vi "Accelerometre 1.vi"() -> ()   [LabVIEW 2019]
uses:
  <vilib>/myRIO/Express VI/Onboard Devices/Accelerometer/Accelerometer Express VI.xnode
  <vilib>/myRIO/Instrument Drivers/Onboard Devices/Accelerometer/vis/Read.vi
  <vilib>/myRIO/Instrument Drivers/Onboard Devices/Accelerometer/Accelerometer.lvlib
  <vilib>/myRIO/Common/Instrument Driver Framework/myRIO v1.0/Accelerometer/typedefs/Accelerometer Channels Enum.ctl
  <vilib>/myRIO/Common/Instrument Driver Framework/myRIO v1.0/Accelerometer/typedefs/Accelerometer Channels List.ctl
  <vilib>/myRIO/Common/Instrument Driver Framework/Utilities/typedefs/Generic FPGA Reference.ctl
  <vilib>/myRIO/Common/Instrument Driver Framework/Utilities/typedefs/myRIO v1.0 Reference.ctl
  <vilib>/myRIO/Common/Instrument Driver Framework/Utilities/typedefs/Hardware Version Enum.ctl
  <vilib>/myRIO/Common/Instrument Driver Framework/Utilities/typedefs/myRIO Generic Hardware Reference.ctl
  <vilib>/myRIO/Instrument Drivers/Onboard Devices/Accelerometer/typedefs/Accelerometer Reference.ctl
  <vilib>/myRIO/Instrument Drivers/Onboard Devices/Accelerometer/vis/myRIO Accelerometer Open.xnode
  <vilib>/myRIO/Common/Instrument Driver Framework/Utilities/vis/Is FPGA Ref Available.vi
  <vilib>/myRIO/Common/Instrument Driver Framework/myRIO v1.0/Accelerometer/vis/myRIO v1.1 Open Accelerometer.vi
  <vilib>/userDefined/High Color/nirio_resource_hc.ctl
  <vilib>/myRIO/Express VI/Onboard Devices/LED/LED Express VI.xnode
  <vilib>/myRIO/Instrument Drivers/Onboard IO/DIO/vis/Write.vi
  <vilib>/myRIO/Instrument Drivers/Onboard IO/DIO/DIO.lvlib
  <vilib>/myRIO/Common/Instrument Driver Framework/myRIO v1.0/DIO/typedefs/DIO Channels Enum.ctl
  <vilib>/myRIO/Common/Instrument Driver Framework/myRIO v1.0/DIO/typedefs/DIO Channels List.ctl
  <vilib>/myRIO/Instrument Drivers/Onboard IO/DIO/typedefs/DIO Reference.ctl
  <vilib>/myRIO/Instrument Drivers/Onboard IO/DIO/vis/myRIO DIO Open.xnode
  <vilib>/myRIO/Common/Instrument Driver Framework/myRIO v1.0/DIO/vis/myRIO v1.1 Open DIO.vi
  Control 1.ctl
panel:
  out "Magnitude":dbl
  in  "stop":bool
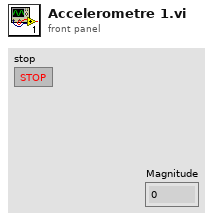
[diagram p1: front panel]
types:
  T1 = typedef "Control 1.ctl" = enum16{"Triggered", "Armed", "Idle"}
  T2 = typedef "DIO.lvlib/DIO Reference.ctl" = cluster{"myRIO Reference":T3, "DIO Channels List":T7}
  T3 = typedef "myRIO Generic Hardware Reference.ctl" = cluster{"myRIO Model":T4, "myRIO Hardware Reference":T5}
  T4 = typedef "Hardware Version Enum.ctl" = enum16{"Unknown", "myRIO-1900", "myRIO-1950", "roboRIO", "NI ELVIS RIO CM", "ELVIS III"}
  T5 = typedef "myRIO v1.0 Reference.ctl" = cluster{"Generic FPGA Reference":T6, "Allow multiple opens":bool}
  T6 = typedef "Generic FPGA Reference.ctl" = refnum<k20>
  T7 = typedef "DIO Channels List.ctl" = T8[]
  T8 = typedef "DIO Channels Enum.ctl" = enum16{"Not Connected", "C/DIO0", "C/DIO1", "C/DIO2", "C/DIO3", "C/DIO4", "C/DIO5", "C/DIO6", "C/DIO7", "A/DIO0", "A/DIO1", "A/DIO2", "A/DIO3", "A/DIO4", "A/DIO5", "A/DIO6", "A/DIO7", "A/DIO8", "A/DIO9", "A/DIO10", "A/DIO11", "A/DIO12", "A/DIO13", "A/DIO14", "A/DIO15", "A/DIO16", "A/DIO17", "A/DIO18", "A/DIO19", "B/DIO0", "B/DIO1", "B/DIO2", "B/DIO3", "B/DIO4", "B/DIO5", "B/DIO6", "B/DIO7", "B/DIO8", "B/DIO9", "B/DIO10", "B/DIO11", "B/DIO12", "B/DIO13", "B/DIO14", "B/DIO15", "B/DIO16", "B/DIO17", "B/DIO18", "B/DIO19", "LED0", "LED1", "LED2", "LED3", "Button0", "DIO/DIO0", "DIO/DIO1", "DIO/DIO2", "DIO/DIO3", "DIO/DIO4", "DIO/DIO5", "DIO/DIO6", "DIO/DIO7", "DIO/DIO8", "DIO/DIO9", "SPI/CS0", "SPI/CS1", "SPI/CS2", "SPI/CS3", "LED RADIO (Green)", "LED RADIO (Red)", "LED COMM (Green)", "LED COMM (Red)", "LED MODE (Green)", "LED MODE (Red)"}
  T9 = typedef "nirio_resource_hc.ctl" = tag
  T10 = typedef "Accelerometer.lvlib/Accelerometer Reference.ctl" = cluster{"myRIO Reference":T3, "Accelerometer Channels List":T11, "LSB Weight":dbl}
  T11 = typedef "Accelerometer Channels List.ctl" = T12[]
  T12 = typedef "Accelerometer Channels Enum.ctl" = enum16{"Not Connected", "X-Axis", "Y-Axis", "Z-Axis"}
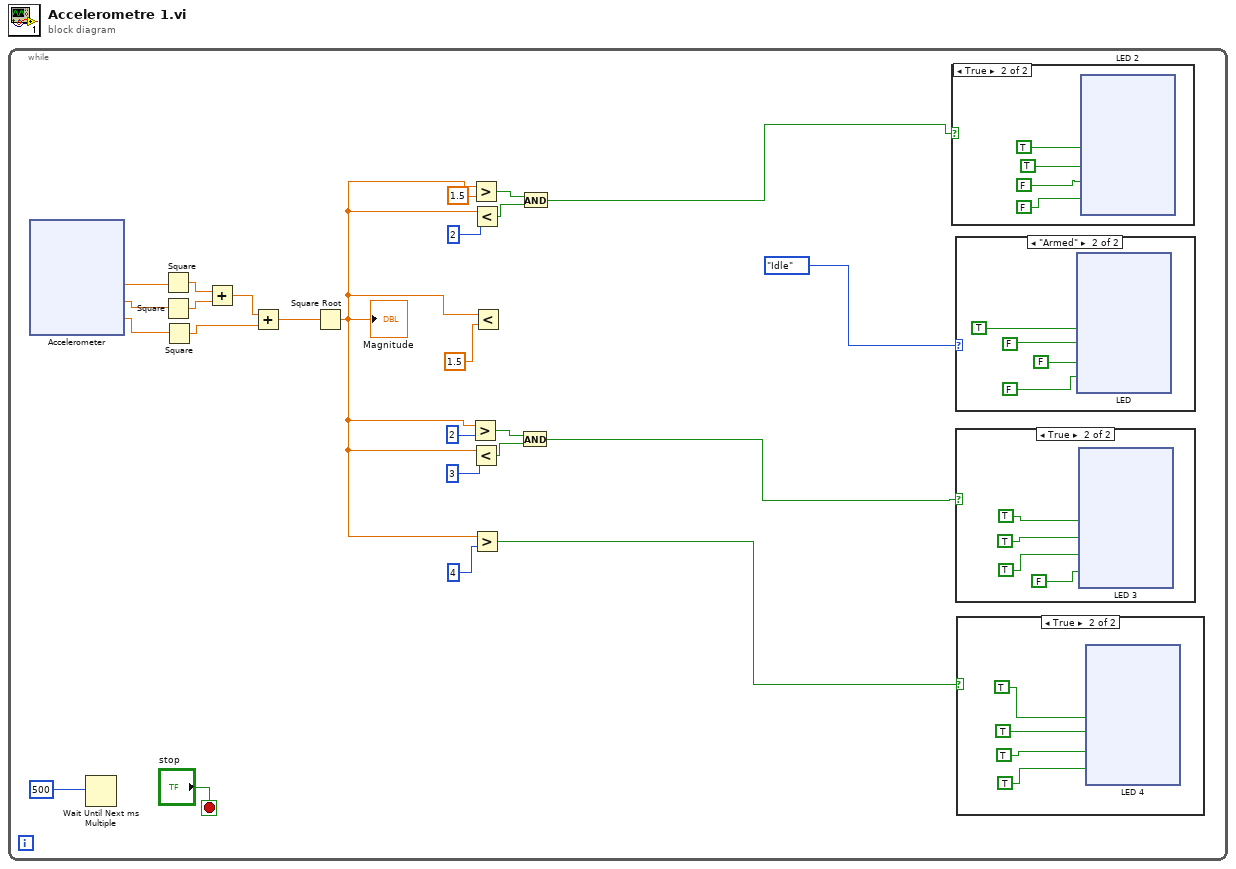
[diagram p0: block diagram]
diagram:
  n1 = while {
    stop <- "stop" stop-if-true
    n2 = xnode "Accelerometer"() -> ("x"=w25:dbl, "y"=w24:dbl, "z"=w23:dbl)  [unwired: 1 in, 1 out]
    n3 = Wait Until Next ms Multiple(millisecond multiple=500) -> ()  [unwired: 1 out]
    n4 = Square(x=w25) -> (x^2=w22:dbl)
    n5 = Square(x=w24) -> (x^2=w21:dbl)
    n6 = Square(x=w23) -> (x^2=w19:dbl)
    n7 = Add(x=w22, y=w21) -> (x+y=w20:dbl)
    n8 = Add(x=w20, y=w19) -> (x+y=w18:dbl)
    n9 = Square Root(x=w18) -> (sqrt(x)=w6:dbl)
    "Magnitude" <- w6
    n10 = Greater?(x=w6, y=2) -> (0:w9:bool)
    n11 = Greater?(x=w6, y=1.5) -> (0:w13:bool)
    n12 = Less?(x=w6, y=3) -> (x < y?=w10:bool)
    n13 = Less?(x=w6, y=2) -> (x < y?=w14:bool)
    n14 = Greater?(x=w6, y=4) -> (0:w3:bool)
    n15 = Less?(x=w6, y=1.5) -> (x < y?=w2:bool)
    n16 = And(x=w9, y=w10) -> (x .and. y?=w4:bool)
    n17 = And(x=w13, y=w14) -> (x .and. y?=w5:bool)
    n18 = case shown="True" w5 {
      frame False {
      }
      frame True {
        n19 = xnode "LED 2"("LED0"=TRUE, "LED1"=TRUE, "LED2"=FALSE, "LED3"=FALSE) -> ()  [unwired: 1 in, 1 out]
      }
    }
    n20 = case shown="\"Armed\"" Control_1."Idle" ("Enum") {
      frame "Triggered", Default {
      }
      frame "Armed" {
        n21 = xnode "LED"("LED0"=TRUE, "LED1"=FALSE, "LED2"=FALSE, "LED3"=FALSE) -> ()  [unwired: 1 in, 1 out]
      }
    }
    n22 = case shown="True" w4 {
      frame False {
      }
      frame True {
        n23 = xnode "LED 3"("LED0"=TRUE, "LED1"=TRUE, "LED2"=TRUE, "LED3"=FALSE) -> ()  [unwired: 1 in, 1 out]
      }
    }
    n24 = case shown="True" w3 {
      frame False {
      }
      frame True {
        n25 = xnode "LED 4"("LED0"=TRUE, "LED1"=TRUE, "LED2"=TRUE, "LED3"=TRUE) -> ()  [unwired: 1 in, 1 out]
      }
    }
  }
